vi "Register for DAQ Events.vi"(8 "error in (no error)":errorcluster, 11 "DAQ Controller in":refnum<class "DAQ Controller.lvclass">) -> (0 "error out":errorcluster, 1 "Process State":refnum<event-registration>, 2 "Daq events":refnum<event-registration>, 3 "DAQ Controller out":refnum<class "DAQ Controller.lvclass">)   [LabVIEW 2022 SP3, in "DAQ Controller.lvclass"]
uses:
  DAQ Controller.lvclass
  DAQ Controller.lvclass/DAQ Controller.ctl
  XY Stage/Process Actor/Process Framework/Process State Data/Process State Data.lvclass
  DAQ Data/DAQ Data.lvclass
  DAQ Data/AIDAQ Data.ctl
  DAQ Data/AI Daq Data.lvlib
  DAQ Data/Events.ctl
  XY Stage/Process Actor/Process Framework/Process State Data/Events.ctl
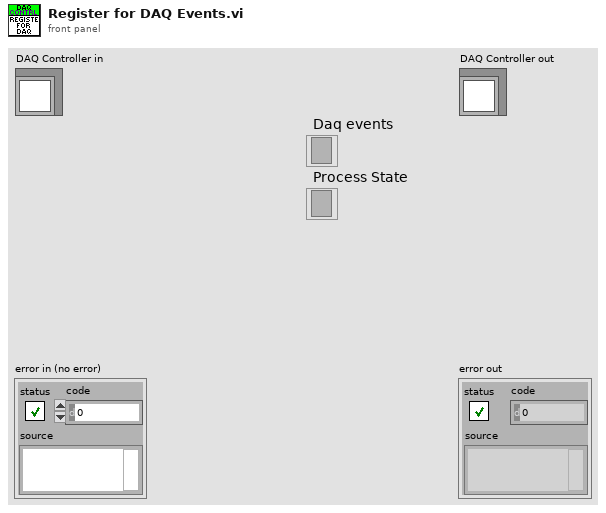
[diagram p1: front panel]
types:
  T1 = typedef "DAQ Data.lvclass/Events.ctl" = cluster{"AI Data":refnum<user-event>, "AI Channel Data":refnum<user-event>}
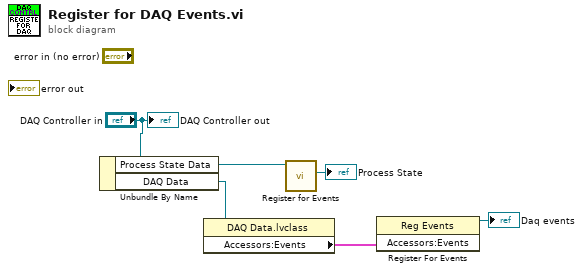
[diagram p0: block diagram]
diagram:
  n1 = Unbundle By Name("DAQ Controller in") -> ("Process State Data"=w5:refnum<data-value>, "DAQ Data"=w4:refnum<data-value>)
  n2 = property class="DAQ Data.lvclass"(reference=w4) -> ("Accessors:Events"=w3:T1)  [unwired: 1 in, 2 out]
  n3 = call "Register for Events.vi"("Process State"=w5) -> ("Event Registration Refnum"=→"Process State":refnum<event-registration>)  [unwired: 8 in, 2 out]
  n4 = register-events(w3) -> (reference out=→"Daq events":refnum<event-registration>)  [unwired: 2 in, 1 out]
  "DAQ Controller out" <- "DAQ Controller in"
